vi "Deserialize Configuration.vi"(8 "error in (no error)":errorcluster, 11 "Serialized Configuration":string) -> (0 "error out":errorcluster, 3 "Configuration":T1)   [LabVIEW 2020, in "ADAS PE Template.lvlib" / "ADAS PE Template.lvclass"]
doc: "<b>Deserailize Configuration</b>\nThis VI is responsible for deserializing the JSON configuration file passed from the <b>Configuration Utility</b>."
uses:
  ADAS PE Template.lvclass
  Configuration.ctl
  <vilib>/ADAS Record/Utilities/ADAS Utilities.lvlib
panel:
  # "#via_ignore"
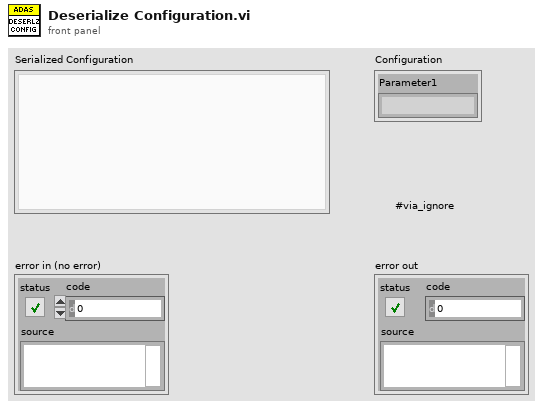
[diagram p1: front panel]
types:
  T1 = typedef "ADAS PE Template.lvlib/ADAS PE Template.lvclass/Configuration.ctl" = cluster{"Parameter1":string}
  T2 = typedef "ADAS Utilities.lvlib/Config Version.ctl" = cluster{"Major":u32, "Minor":u32, "Fix":u32, "Build":u32}
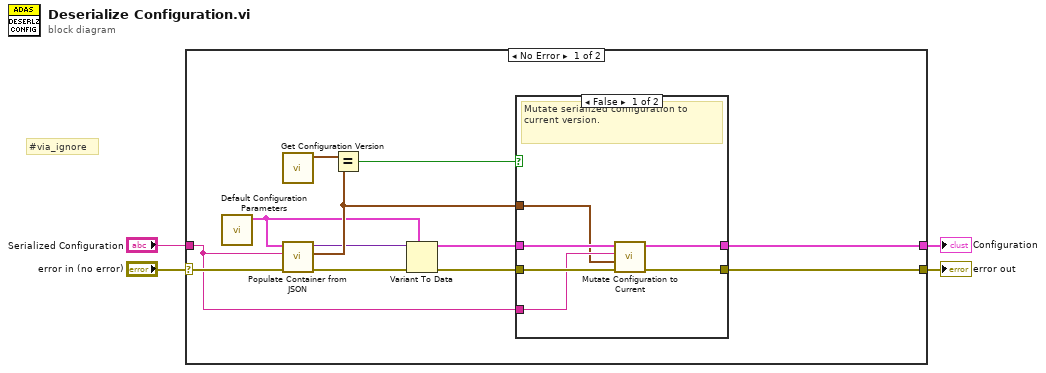
[diagram p0: block diagram]
diagram:
  # "#via_ignore"
  n1 = case shown="No Error" "error in (no error)" {
    selector: "error in (no error)" -> [w14 w25]
    tunnel: [w10 w25] -> w3
    tunnel: [w11 _] -> w2
    tunnel: "Serialized Configuration" -> [w12 _]
    frame No Error {
      n2 = call "Default Configuration Parameters.vi"() -> ("Default Configuration"=w5:T1)  [unwired: 11 in]
      n3 = call "Get Configuration Version.vi"() -> ("Version"=w16:T2)  [unwired: 11 in]
      n4 = call <vilib>:"Populate Container from JSON.vi"("error in (no error)"=w14, "JSON string In"=w12, "Container In"=w5) -> ("error out"=w9:errorcluster, "Version Out"=w13:T2, "Container Out"=w7:variant)  [unwired: 6 in]
      n5 = Equal?(x=w16, y=w13) -> (x = y?=w15:bool)
      n6 = Variant To Data(error in=w9, type=w5, Variant=w7) -> (data=w6:T1, error out=w8:errorcluster)
      n7 = case shown="False" w15 {
        tunnel: w8 -> [w20 w23]
        tunnel: [w22 w23] -> w10
        tunnel: [w21 w24] -> w11
        tunnel: w13 -> [w17 _]
        tunnel: w12 -> [w18 _]
        tunnel: w6 -> [w19 w24]
        frame False {
          # "Mutate serialized configuration to current version."
          n8 = call "Mutate Configuration to Current.vi"("error in (no error)"=w20, "Serialized Version"=w17, "Serialized Configuration in"=w18, "Automated Config Attempt"=w19) -> ("error out"=w22:errorcluster, "Config Out"=w21:T1)  [unwired: 6 in]
        }
        frame True {
          # "Already the current version"
        }
      }
    }
    frame Error {
    }
  }
  "Configuration" <- w2
  "error out" <- w3
